vi "Run Test - Pause Condition (SubVI).vi"(8 "error in (no error)":errorcluster, 11 "Cluster in":T1 {"M Event" items=["Stop", "Running", "PID", "Up Limit", "Down Limit", "Load Limit"]; "Test Type" items=["Please Select", "Triaxial Shear", "Triaxial UU", "Shearbox", "Permeability", "Consolidation (Stepped Loading)/Swelling", "Saturation (Incremental)", "User Defined", "UCT", "Isotropic Consolidation", "Swelling Pressure"]; "Data"."Test Type" items=["Please Select", "Triaxial Shear", "Triaxial UU", "Shearbox", "Permeability", "Consolidation (Stepped Loading)/Swelling", "Saturation (Incremental)", "User Defined", "UCT", "Isotropic Consolidation", "Swelling Pressure"]}) -> (0 "error out":errorcluster, 3 "Cluster out":T1 {"M Event" items=["Stop", "Running", "PID", "Up Limit", "Down Limit", "Load Limit"]; "Test Type" items=["Please Select", "Triaxial Shear", "Triaxial UU", "Shearbox", "Permeability", "Consolidation (Stepped Loading)/Swelling", "Saturation (Incremental)", "User Defined", "UCT", "Isotropic Consolidation", "Swelling Pressure"]; "Data"."Test Type" items=["Please Select", "Triaxial Shear", "Triaxial UU", "Shearbox", "Permeability", "Consolidation (Stepped Loading)/Swelling", "Saturation (Incremental)", "User Defined", "UCT", "Isotropic Consolidation", "Swelling Pressure"]})   [LabVIEW 2019]
uses:
  Controls/RunTest - Data Structure.ctl
  Controls/Test Panel - Data Structure.ctl
  Controls/Station - Test Type.ctl
  <vilib>/Utility/miscctls.llb/LVRowAndColumnTypeDef.ctl
  Controls/RunTest - Calculate Data.ctl
  <vilib>/httpClient/ClientHandle.ctl
  Controls/RunTest - Start Condition.ctl
  Controls/RunTest - Stop Condition.ctl
  Controls/UDP - Event.ctl
  Controls/RunTest - State.ctl
  Controls/UDP - Command.ctl
  <vilib>/httpClient/LabVIEWHTTPClient.lvlib
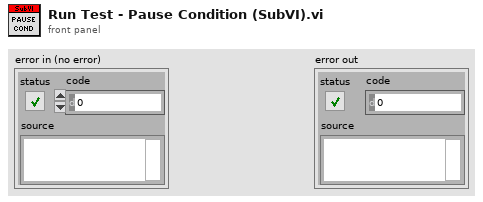
[diagram p1: front panel]
types:
  T1 = typedef "RunTest - Data Structure.ctl" = cluster{"Test Plan":string[], "PlanRow":i32, "Device Name":string[], "Timeout":i32, "Start?":bool, "Pause?":bool, "IP Address":string[], "LogRow":i32, "Logtype":u16, "Log Elapse":sgl, "Data":T2, "Stop log?":bool, "tdms":refnum<k34>, "Sensor Data":sgl[], "Start time":timestamp, "Prev Log Elapse":u32, "Plot":u16, "X-Axis":u16[], "Y-Axis":u16[], "XY":cluster{"X":dbl, "Y":dbl}[][], "End Stage?":bool, "1run":bool, "Condition":u16[], "Start Con":bool, "Log Con":bool, "Stop Con":bool, "Start Elapse":dbl, "Start Load":dbl, "Motor":i32, "StartRow":i32, "number log":i32, "Dir":bool, "Start time test":timestamp, "Auto":bool, "Check return?":bool, "Inv":cluster{"M":i32[], "Bool":bool[]}, "tdms temp":refnum<k34>, "Zero?":bool, "Plot Timer":dbl, "1st Run":bool, "TDMS Path":path, "MaxLoad":dbl, "Log Timer":sgl[], "Test Type":T3, "Log Sensor":string[], "Save?":bool, "1st Log":bool, "Y-Axis 2":u16[], "On Y-Axis 2":bool, "Decimal":u8[], "Init":cluster{"PWP TS":sgl, "Load TS":sgl, "Volume TS":sgl, "Disp TS":sgl, "CP":sgl, "Vol In":sgl, "Vol Out":sgl, "Load UCT":sgl, "Disp UCT":sgl, "PWP Sat":sgl, "CP Sat":sgl, "Volume IsoCons":sgl, "PWP IsoCons":sgl, "PWP TUU":sgl, "Load TUU":sgl, "Volume TUU":sgl, "Disp TUU":sgl, "Load Cons":sgl, "Disp Cons":sgl, "Volume Sat":sgl, "Vertical Load SB":sgl, "Vertical Disp SB":sgl, "H Disp SB":sgl, "H Load SB":sgl}, "Calc":T5, "Device Index":i32[], "Channel Index":i32[], "http ref":T6, "fileid":string, "Step Cons":cluster{"V Stress":sgl, "H Settlement":sgl}, "RunTest":bool, "Graph Last":i32, "Init?":bool, "Datalog":bool[], "Start":T7, "Stop":T8, "Running?":bool, "StartTime":dbl, "Log Prev Time":dbl, "KeyName":string[], "Test RunTime":dbl, "Log Prev Axial":dbl, "M Event":T9[], "Last Log":bool, "popup":bool, "PreStart UU":bool, "PreStart Sat":bool}
  T2 = typedef "Test Panel - Data Structure.ctl" = cluster{"Station":string, "Sample ID":string, "Job No":string, "Job Description":string, "Filename":string, "Test Type":T3, "Speciment No":string, "Depth":string, "Height":string, "Diameter/Length":string, "Weight":string, "Test Parameter":string, "Station[]":string[], "Edit Pos":T4, "Edit Pos Prev":T4, "Area":string, "Path":string}
  T3 = typedef "Station - Test Type.ctl" = u16
  T4 = typedef "LVRowAndColumnTypeDef.ctl" = cluster{"Row":i32, "Column":i32}
  T5 = typedef "RunTest - Calculate Data.ctl" = cluster{"TS":cluster{"Change PWP":sgl, "Change Vol":sgl, "Axial Load":sgl, "CiL":sgl, "Deviator":sgl, "Axial Strain":sgl, "MaxDeviator":sgl}, "TUU":cluster{"Change PWP":sgl, "Axial Load":sgl, "CiL":sgl, "Deviator":sgl, "Axial Strain":sgl, "MaxDeviator":sgl}, "Sat":cluster{"B Value":sgl, "PWP Diss":sgl, "CPP":sgl, "CV":sgl}, "Per":cluster{"Change Vol In":sgl, "Change Vol Out":sgl, "Mean Vol":sgl, "Gradient Pressure":sgl, "Outlet Flow":sgl, "Inlet Flow":sgl, "I X1":sgl, "I X2":sgl, "I Y1":sgl, "I Y2":sgl, "O X1":sgl, "O X2":sgl, "O Y1":sgl, "O Y2":sgl}, "Step Cons":cluster{"V Stress":sgl, "H Settlement":sgl, "Total H Settle":sgl, "Prev Total H":sgl}, "UCT":cluster{"ALC":sgl, "H Change":sgl, "Deviator":sgl, "Axial Strain":sgl, "V Stress":sgl, "MaxDeviator":sgl}, "ISO Cons":cluster{"CPP":sgl, "PWP Diss":sgl, "CV":sgl}, "SB":cluster{"Speci LenC":sgl, "Shear Strain":sgl, "H LC":sgl, "Normal Stress":sgl, "Shear Stress":sgl, "MaxShear":sgl}}
  T6 = typedef "LabVIEWHTTPClient.lvlib/ClientHandle.ctl" = refnum<k1>
  T7 = typedef "RunTest - Start Condition.ctl" = cluster{"Cons":cluster{"VS":dbl, "Delay":bool, "No Delay":dbl}, "Sat":cluster{"CP":dbl, "BP":dbl, "StartBP":bool, "Target CP":bool, "Target BP":bool}, "Iso":cluster{"BP":dbl}, "TS":cluster{"SS":dbl, "Engage":bool, "ES":dbl, "LC":dbl, "PreStart":bool, "Trig SS":bool, "Drain":dbl}, "TUU":cluster{"SS":dbl, "Engage":bool, "ES":dbl, "LC":dbl, "PreStart":bool, "Trig SS":bool, "CP":dbl, "Delay Value":dbl, "Delay":bool, "CP PID":bool}, "UCT":cluster{"SS":dbl, "Engage":bool, "ES":dbl, "LC":dbl, "PreStart":bool, "Trig SS":bool}, "Enable?":bool, "SB":cluster{"SS":dbl, "Engage":bool, "ES":dbl, "LC":dbl, "PreStart":bool, "Trig SS":bool, "VS":dbl, "Delay Value":dbl, "Delay":bool, "VS PID":bool}, "Perm":cluster{"DP":dbl}}
  T8 = typedef "RunTest - Stop Condition.ctl" = cluster{"Cons":cluster{"Select":i32, "Disp":dbl, "Time":dbl, "Time2":dbl, "Disp 2":dbl, "Time Cond":dbl, "Last Disp":dbl, "Swell":bool}, "Sat":cluster{"Select":i32, "PP":dbl, "Time":dbl, "VC":dbl, "Time2":dbl, "Time Cond":dbl, "Last PP":dbl, ".B":bool, "B":dbl, "Last Vc":dbl, "Time Cond 2":dbl, "Time3":dbl, "Time Cond 3":dbl}, "Iso":cluster{"PP":dbl, "Time":dbl, "VC":dbl, "Time2":dbl, "Time Cond":dbl, "Last Vc":dbl, ".PP":bool, "Time Cond 2":dbl, "Select":i32}, "TS":cluster{"Axial":dbl, ".MaxDev":bool, "MaxDev Value":dbl, "Return":bool, "Reset":bool, "Prev Time":dbl, "PostStop Run":bool, "CP Stop":bool, "BP Stop":bool, "PostStop Trig":bool, "Reset Value":dbl, "BPTrig":bool, "CPTrig":bool, "VLCTrig":bool}, "TUU":cluster{"Axial":dbl, ".MaxDev":bool, "MaxDev Value":dbl, "Return":bool, "Reset":bool, "Prev Time":dbl, "PostStop Run":bool, "CP Stop":bool, "BP Stop":bool, "PostStop Trig":bool, "Reset Value":dbl, "BPTrig":bool, "CPTrig":bool, "VLCTrig":bool}, "UCT":cluster{"Axial":dbl, ".MaxDev":bool, "MaxDev Value":dbl, "Return":bool, "Reset":bool, "Prev Time":dbl, "PostStop Run":bool, "CP Stop":bool, "BP Stop":bool, "PostStop Trig":bool}, "Enable?":bool, "SB":cluster{"Shear":dbl, ".MaxShear":bool, "MaxShear Value":dbl, "Return":bool, "Reset":bool, "Prev Time":dbl, "PostStop Run":bool, "CP Stop":bool, "BP Stop":bool, "PostStop Trig":bool, "Reset Value":dbl, "BPTrig":bool, "CPTrig":bool, "VLCTrig":bool}, "Perm":cluster{"Max Time":bool, "Reset":bool, "PostStop Run":bool, "Ratio":bool, "Reset Value":dbl, "Time":dbl, "RatioTime":dbl, "RatioMore":dbl, "RatioLess":dbl, "Time Cond":dbl, "Time Cond 2":dbl, "Prev IF":dbl, "Prev OF":dbl, "PostStop Trig":bool, "BP Trig":bool, "DP Stop":bool, "BP Stop":bool, "CP Stop":bool, "CP Trig":bool}, "SP":cluster{".Max Time":bool, ".Time":bool, "Time":dbl, "MaxTime":dbl, "Time Cond":dbl, "Max Time Cond":dbl, "Stress":dbl}}
  T9 = typedef "UDP - Event.ctl" = u16
  T10 = enum32{"Please Select", "Triaxial Shear", "Triaxial UU", "Shearbox", "Permeability", "Consolidation", "Saturation", "User Defined", "UCT", "Iso Consolidation"}
  T11 = typedef "UDP - Command.ctl" = enum16{"Stop", "Jog Up", "Jog Down", "Ramp Up", "Ramp Down", "PID Target", "PID Ramp", "Disp Run", "Read Ch Data", "Zero Channel", "Zero Disp", "Read Sensor", "Write Sensor", "Read ADC", "Write ADC", "Read PID", "Write PID", "Read Test", "Write Test", "Read System", "Write System", "Read Datalog", "Read Datalog Sensor"}
  T12 = typedef "RunTest - State.ctl" = enum16{"Load Testfile", "Notifier", "Init", "Idle", "Load", "Read DB", "Run", "Pause", "Stop", "Check Start", "Check Stop", "Check Post Stop", "Check Log", "EndStage", "Data View", "Display", "Graph", "Graph Old", "Close", "Stop PID", "Check Limit", "Auto", "Up", "Log", "Zero", "Machine Control", "Save Report"}
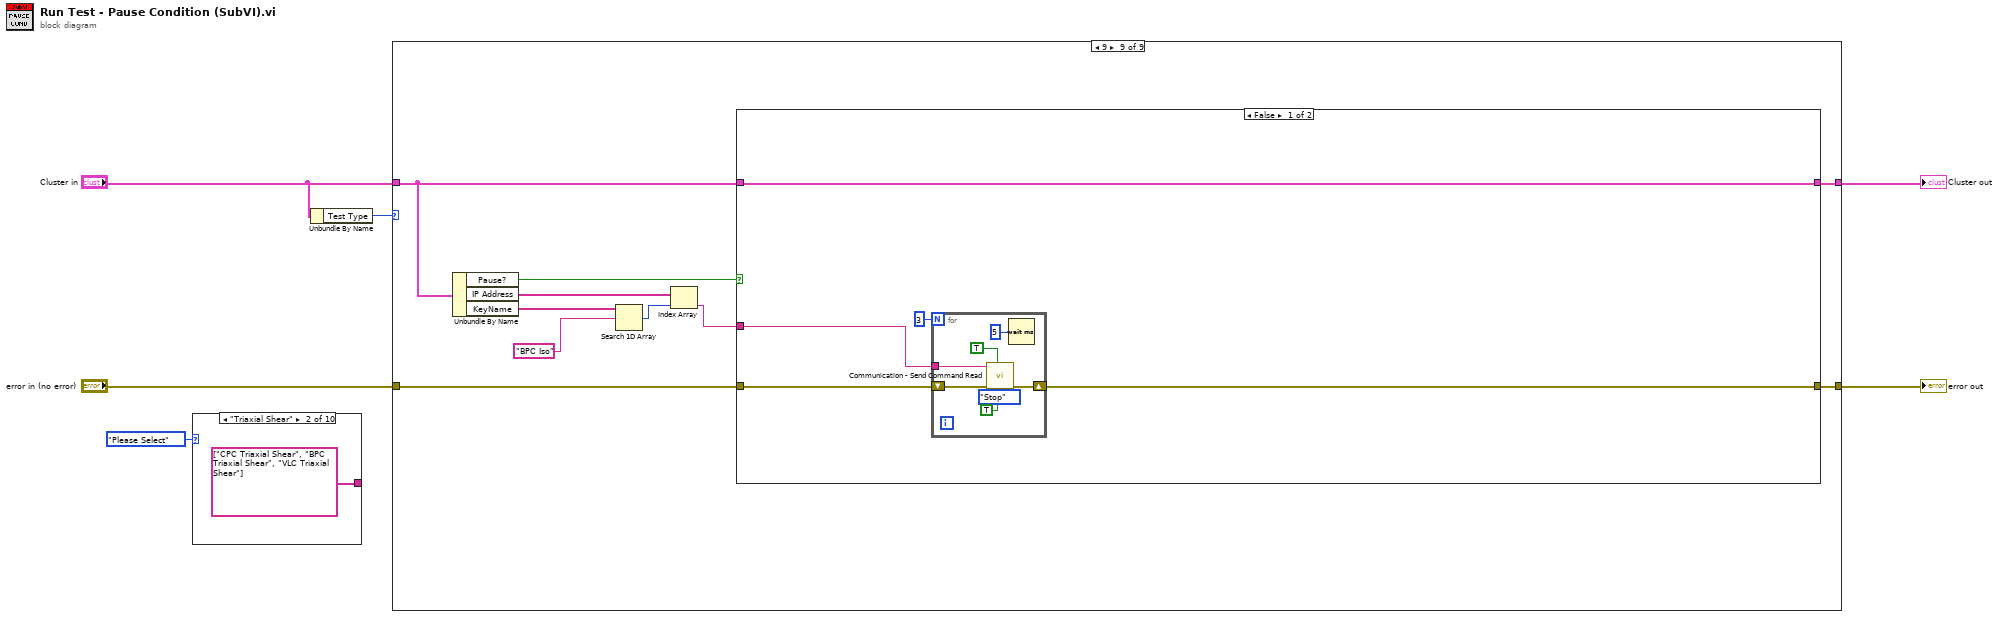
[diagram p0: block diagram]
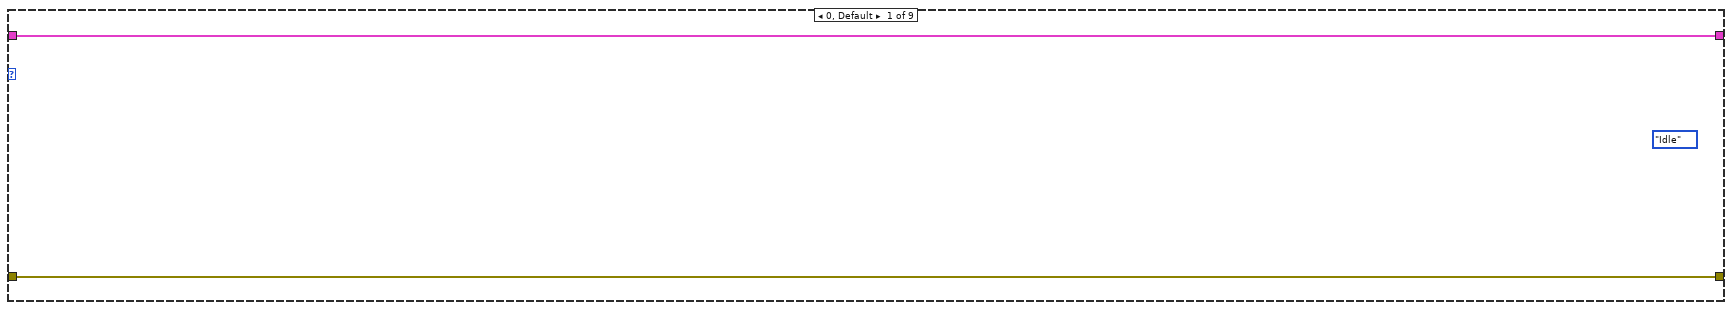
[diagram p2: hidden frame]
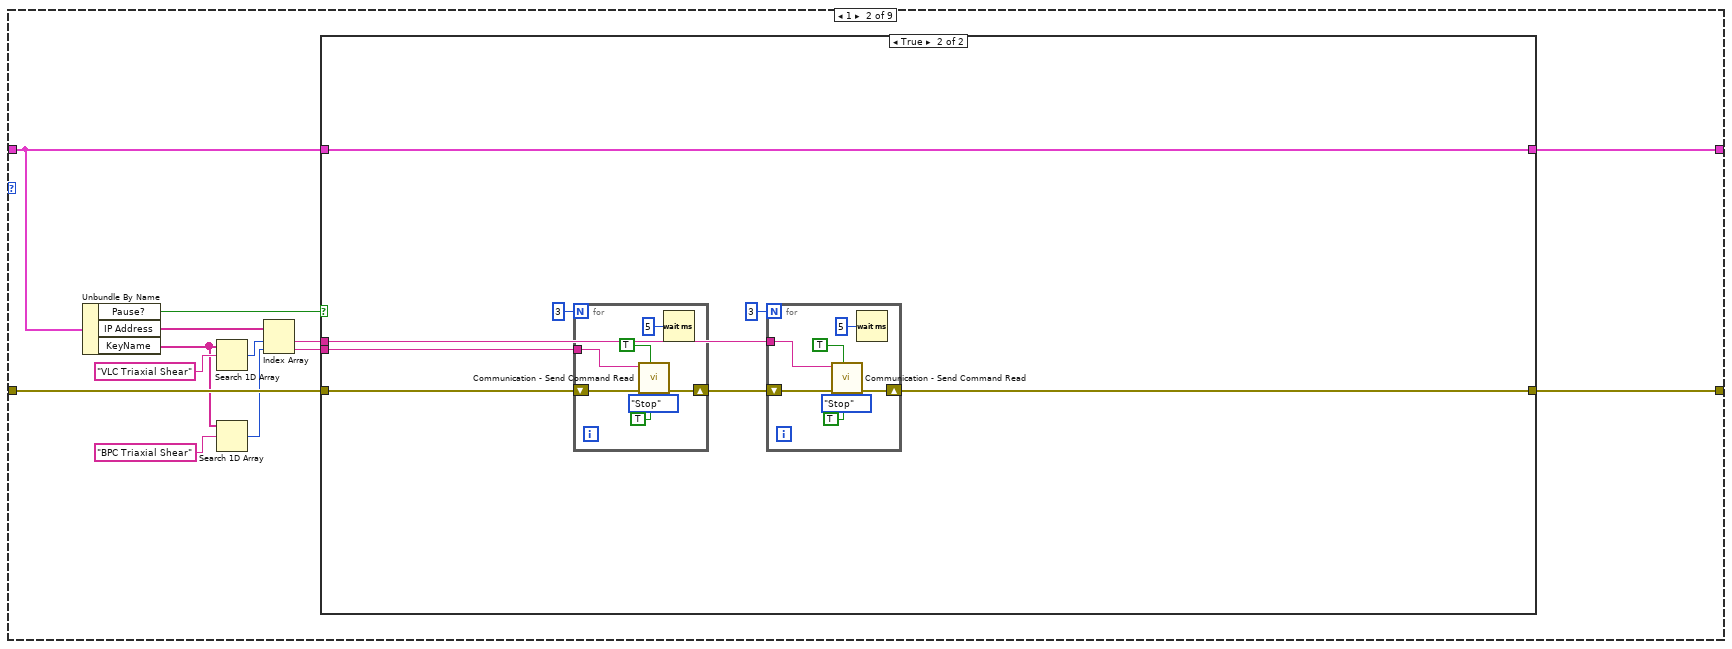
[diagram p3: hidden frame]
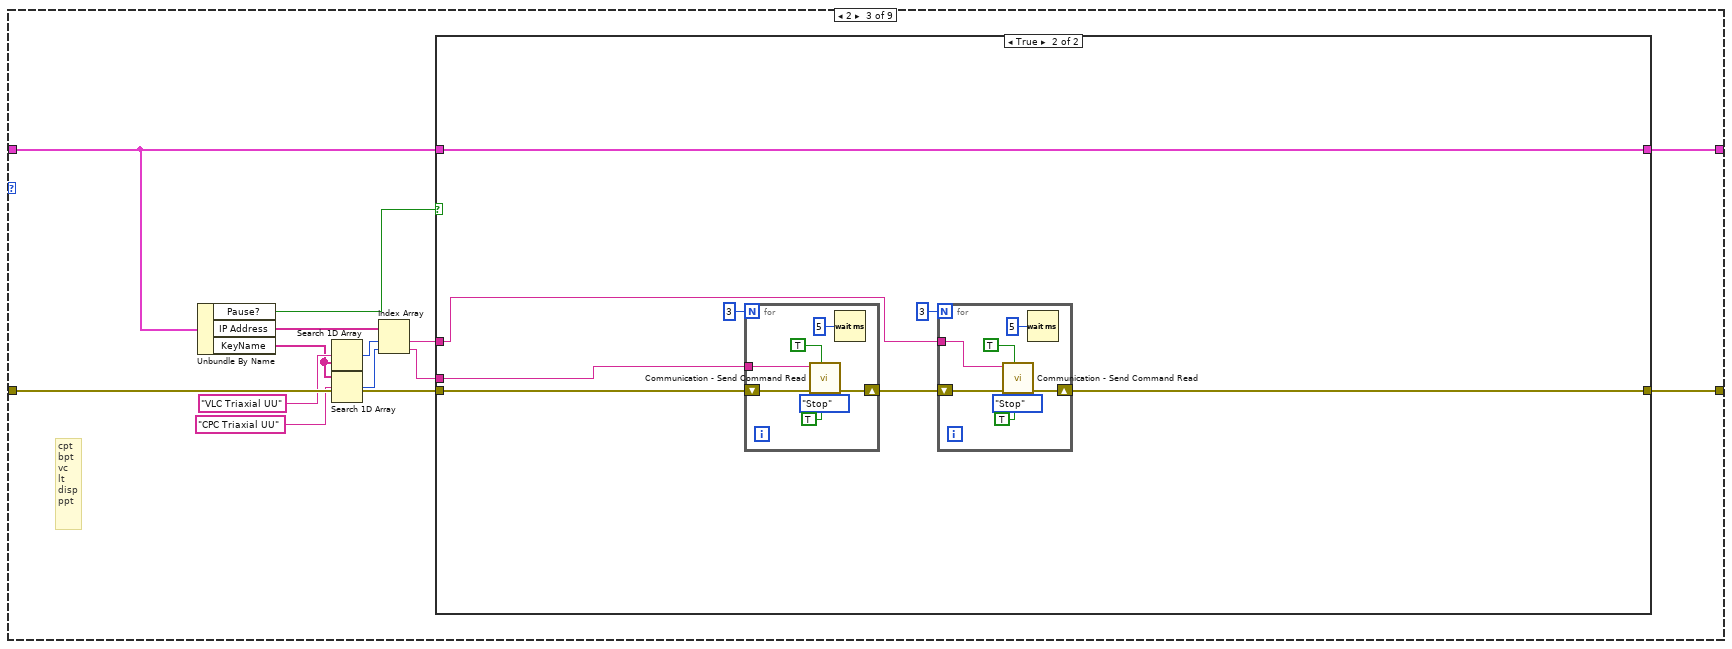
[diagram p5: hidden frame]
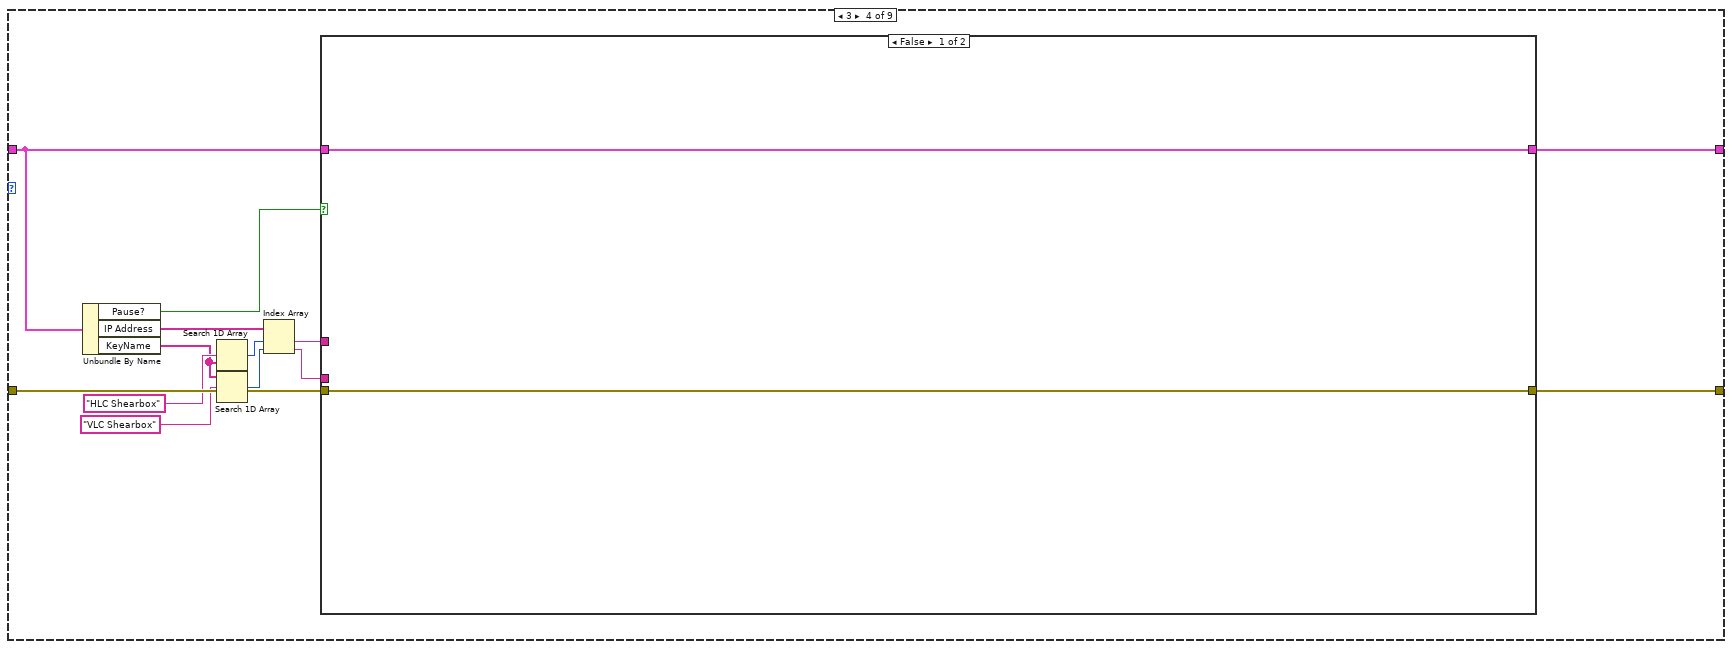
[diagram p7: hidden frame]
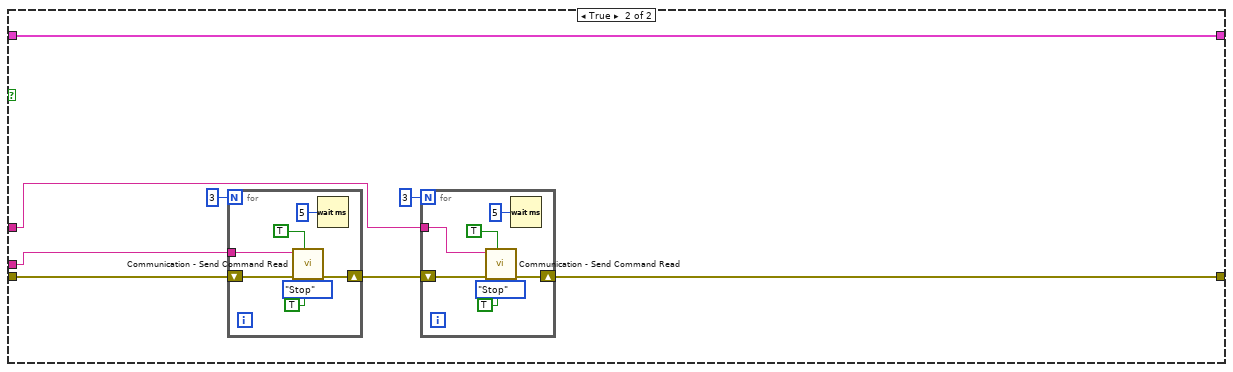
[diagram p8: hidden frame]
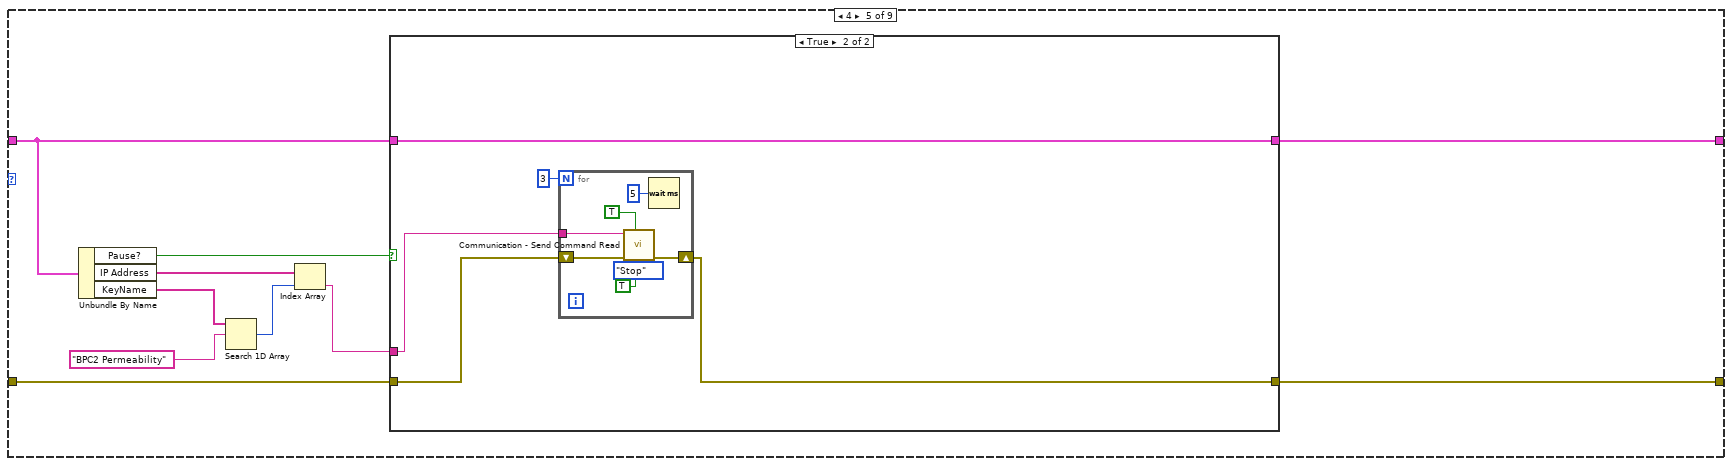
[diagram p9: hidden frame]
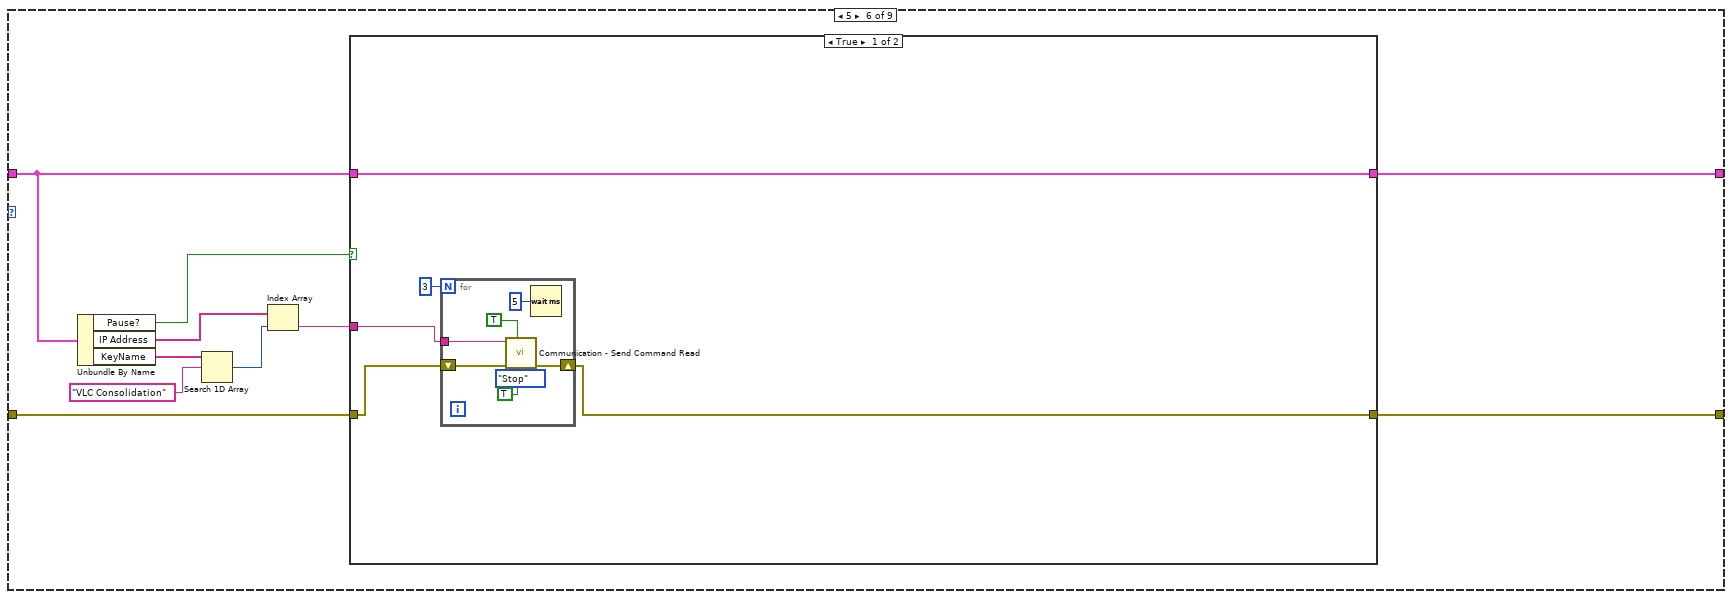
[diagram p11: hidden frame]
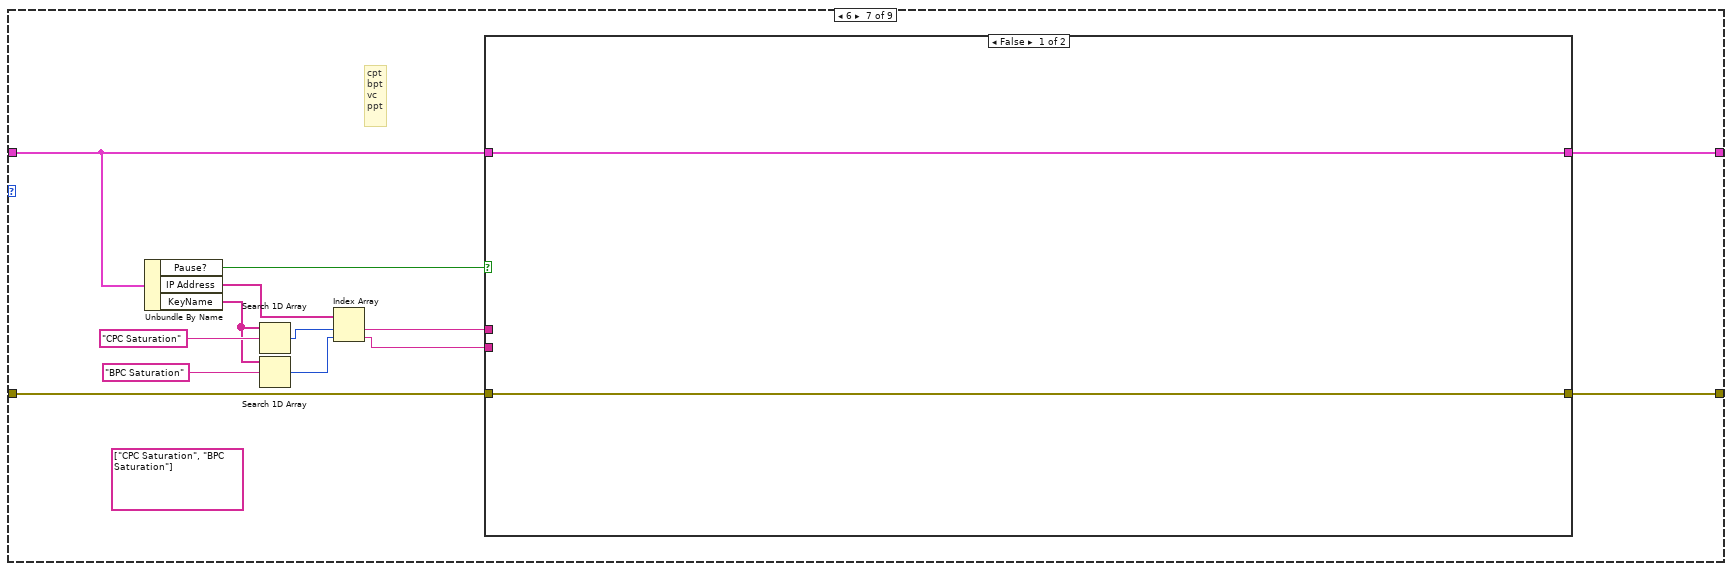
[diagram p13: hidden frame]
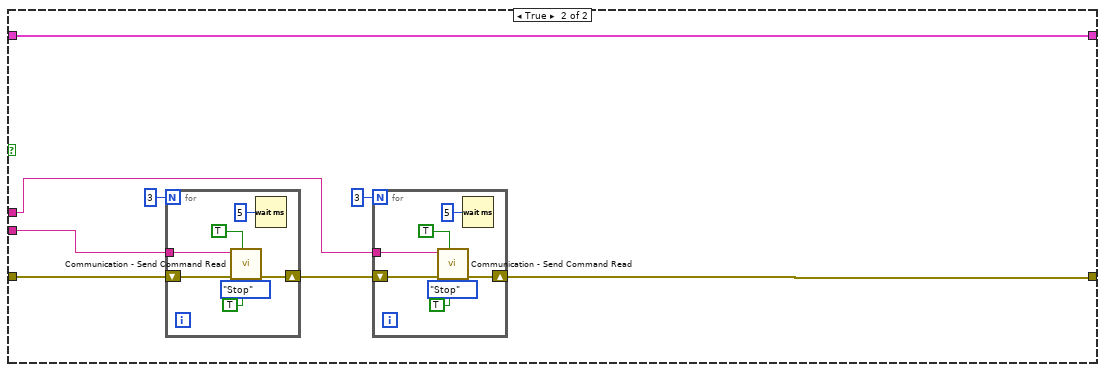
[diagram p14: hidden frame]
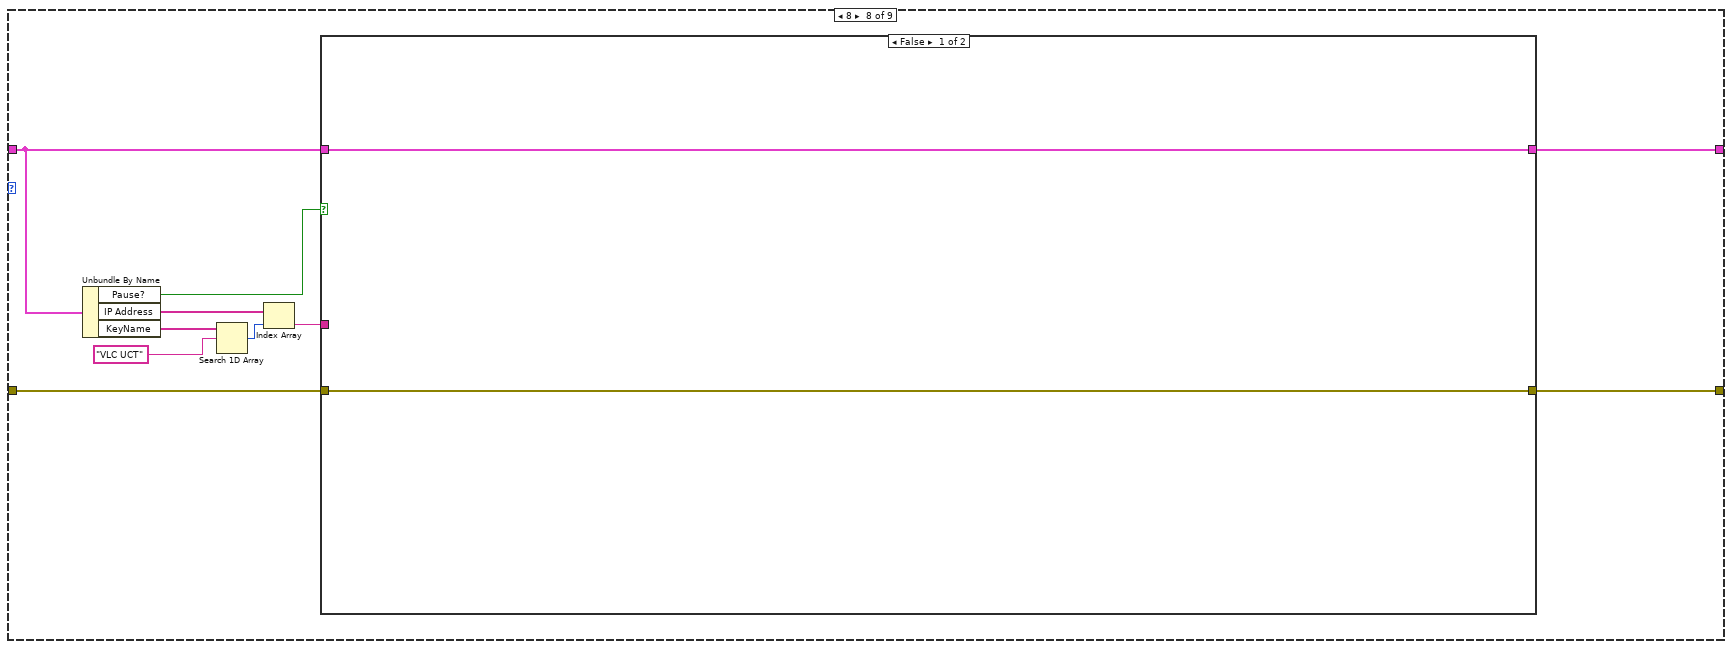
[diagram p15: hidden frame]
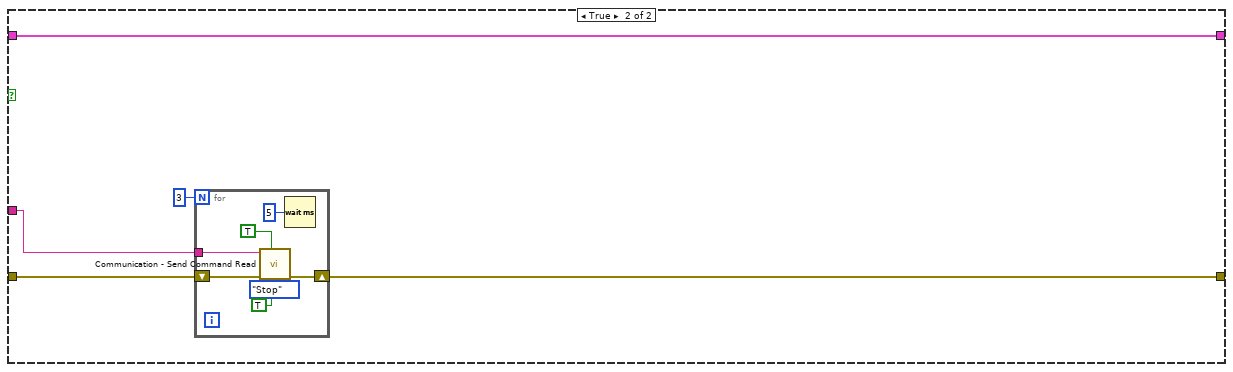
[diagram p16: hidden frame]
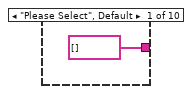
[diagram p18: hidden frame]
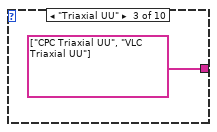
[diagram p19: hidden frame]
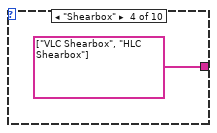
[diagram p20: hidden frame]
diagram:
  n1 = case shown="\"Triaxial Shear\"" T10."Please Select" ("Sub Tab") {
    tunnel: [string[] [] string[] ["CPC Triaxial Shear", "BPC Triaxial Shear", "VLC Triaxial Shear"] string[] ["CPC Triaxial UU", "VLC Triaxial UU"] string[] ["VLC Shearbox", "HLC Shearbox"] string[] ["CPC Permeability", "BPC Permeability", "BPC2 Permeability"] string[] ["VLC Consolidation"] string[] ["CPC Saturation", "BPC Saturation"] string[] ["CPC User Defined", "BPC User Defined", "BPC2 User Defined", "VLC User Defined", "HLC User Defined"] string[] ["VLC UCT"] string[] ["CPC Iso", "BPC Iso"]] -> _
    frame "Please Select", Default {
    }
    frame "Triaxial Shear" {
    }
    frame "Triaxial UU" {
    }
    frame "Shearbox" {
    }
    frame "Permeability" {
    }
    frame "Consolidation" {
    }
    frame "Saturation" {
    }
    frame "User Defined" {
    }
    frame "UCT" {
    }
    frame "Iso Consolidation" {
    }
  }
  n2 = Unbundle By Name("Cluster in") -> ("Test Type"=w1:T3)
  n3 = case shown="9" w1 {
    tunnel: [w18 w29 w67 w94 w136 w161 w188 w222 w245] -> w3
    tunnel: "Cluster in" -> [w18 w30 w65 w104 w135 w160 w187 w223 w244]
    tunnel: [w17 w28 w66 w95 w139 w163 w190 w221 w248] -> w5
    tunnel: "error in (no error)" -> [w17 w31 w68 w105 w138 w162 w189 w224 w247]
    frame 0, Default {
      (unwired) RunTest_-_State."Idle"
    }
    frame 1 {
      n4 = Unbundle By Name(w30) -> ("Pause?"=w19:bool, "IP Address"=w26:string[], "KeyName"=w22:string[])
      n5 = Search 1D Array(1D array=w22, element="VLC Triaxial Shear" ("String")) -> (index of element=w27:i32)  [unwired: 1 in]
      n6 = Search 1D Array(1D array=w22, element="BPC Triaxial Shear" ("String")) -> (index of element=w21:i32)  [unwired: 1 in]
      n7 = Index Array(array=w26, index #1=w27, index #2=w21) -> (element #1=w24:string, element #2=w20:string)
      n8 = case shown="True" w19 {
        tunnel: w31 -> [w33 w41]
        tunnel: w30 -> [w32 w40]
        tunnel: [w32 w40] -> w29
        tunnel: [w33 w35] -> w28
        tunnel: w24 -> [_ w34]
        tunnel: w20 -> [_ w39]
        frame False {
        }
        frame True {
          n9 = for {
            N: 3 -> [_]
            tunnel: w39 -> [w50]
            shift-right: [w51] -> w36
            shift-left: w41 -> [w52]
            n10 = call "Communication - Send Command Read.vi"("Fron?"=TRUE, "Bypass?"=TRUE, "error in (no error)"=w52, "Action"=UDP_-_Command."Stop", "Device IP Address"=w50) -> ("error out"=w51:errorcluster)  [unwired: 6 in]
            n11 = Wait (ms)(milliseconds to wait=u32 5) -> ()  [unwired: 1 out]
          }
          n12 = for {
            N: 3 -> [_]
            tunnel: w34 -> [w43]
            shift-right: [w44] -> w35
            shift-left: w36 -> [w45]
            n13 = call "Communication - Send Command Read.vi"("Fron?"=TRUE, "Bypass?"=TRUE, "error in (no error)"=w45, "Action"=UDP_-_Command."Stop", "Device IP Address"=w43) -> ("error out"=w44:errorcluster)  [unwired: 6 in]
            n14 = Wait (ms)(milliseconds to wait=u32 5) -> ()  [unwired: 1 out]
          }
        }
      }
    }
    frame 2 {
      # "cpt\nbpt\nvc\nlt\ndisp\nppt"
      n15 = Unbundle By Name(w65) -> ("Pause?"=w56:bool, "IP Address"=w63:string[], "KeyName"=w60:string[])
      n16 = Search 1D Array(1D array=w60, element="VLC Triaxial UU" ("String")) -> (index of element=w64:i32)  [unwired: 1 in]
      n17 = Search 1D Array(1D array=w60, element="CPC Triaxial UU" ("String")) -> (index of element=w58:i32)  [unwired: 1 in]
      n18 = Index Array(array=w63, index #1=w64, index #2=w58) -> (element #1=w61:string, element #2=w57:string)
      n19 = case shown="True" w56 {
        tunnel: w68 -> [w69 w74]
        tunnel: w65 -> [w70 w78]
        tunnel: [w70 w78] -> w67
        tunnel: [w69 w73] -> w66
        tunnel: w61 -> [_ w71]
        tunnel: w57 -> [_ w72]
        frame False {
        }
        frame True {
          n20 = for {
            N: 3 -> [_]
            shift-right: [w88] -> w75
            shift-left: w74 -> [w89]
            tunnel: w72 -> [w86]
            n21 = call "Communication - Send Command Read.vi"("Fron?"=TRUE, "Bypass?"=TRUE, "error in (no error)"=w89, "Action"=UDP_-_Command."Stop", "Device IP Address"=w86) -> ("error out"=w88:errorcluster)  [unwired: 6 in]
            n22 = Wait (ms)(milliseconds to wait=u32 5) -> ()  [unwired: 1 out]
          }
          n23 = for {
            N: 3 -> [_]
            tunnel: w71 -> [w80]
            shift-right: [w81] -> w73
            shift-left: w75 -> [w82]
            n24 = call "Communication - Send Command Read.vi"("Fron?"=TRUE, "Bypass?"=TRUE, "error in (no error)"=w82, "Action"=UDP_-_Command."Stop", "Device IP Address"=w80) -> ("error out"=w81:errorcluster)  [unwired: 6 in]
            n25 = Wait (ms)(milliseconds to wait=u32 5) -> ()  [unwired: 1 out]
          }
        }
      }
    }
    frame 3 {
      n26 = Unbundle By Name(w104) -> ("Pause?"=w93:bool, "IP Address"=w102:string[], "KeyName"=w99:string[])
      n27 = Search 1D Array(1D array=w99, element="HLC Shearbox" ("String")) -> (index of element=w103:i32)  [unwired: 1 in]
      n28 = Search 1D Array(1D array=w99, element="VLC Shearbox" ("String")) -> (index of element=w97:i32)  [unwired: 1 in]
      n29 = Index Array(array=w102, index #1=w103, index #2=w97) -> (element #1=w100:string, element #2=w96:string)
      n30 = case shown="False" w93 {
        tunnel: w105 -> [w106 w112]
        tunnel: w104 -> [w107 w110]
        tunnel: w100 -> [_ w108]
        tunnel: w96 -> [_ w109]
        tunnel: [w106 w111] -> w95
        tunnel: [w107 w110] -> w94
        frame False {
        }
        frame True {
          n31 = for {
            N: 3 -> [_]
            shift-right: [w125] -> w113
            shift-left: w112 -> [w126]
            tunnel: w109 -> [w123]
            n32 = call "Communication - Send Command Read.vi"("Fron?"=TRUE, "Bypass?"=TRUE, "error in (no error)"=w126, "Action"=UDP_-_Command."Stop", "Device IP Address"=w123) -> ("error out"=w125:errorcluster)  [unwired: 6 in]
            n33 = Wait (ms)(milliseconds to wait=u32 5) -> ()  [unwired: 1 out]
          }
          n34 = for {
            N: 3 -> [_]
            tunnel: w108 -> [w117]
            shift-right: [w118] -> w111
            shift-left: w113 -> [w119]
            n35 = call "Communication - Send Command Read.vi"("Fron?"=TRUE, "Bypass?"=TRUE, "error in (no error)"=w119, "Action"=UDP_-_Command."Stop", "Device IP Address"=w117) -> ("error out"=w118:errorcluster)  [unwired: 6 in]
            n36 = Wait (ms)(milliseconds to wait=u32 5) -> ()  [unwired: 1 out]
          }
        }
      }
    }
    frame 4 {
      n37 = Unbundle By Name(w135) -> ("Pause?"=w137:bool, "IP Address"=w132:string[], "KeyName"=w134:string[])
      n38 = Search 1D Array(1D array=w134, element="BPC2 Permeability" ("String")) -> (index of element=w131:i32)  [unwired: 1 in]
      n39 = Index Array(array=w132, index=w131) -> (element=w130:string)
      n40 = case shown="True" w137 {
        tunnel: [w141 w143] -> w139
        tunnel: w138 -> [w141 w144]
        tunnel: [w140 w146] -> w136
        tunnel: w135 -> [w140 w146]
        tunnel: w130 -> [_ w142]
        frame False {
        }
        frame True {
          n41 = for {
            N: 3 -> [_]
            shift-right: [w149] -> w143
            shift-left: w144 -> [w150]
            tunnel: w142 -> [w147]
            n42 = call "Communication - Send Command Read.vi"("Fron?"=TRUE, "Bypass?"=TRUE, "error in (no error)"=w150, "Action"=UDP_-_Command."Stop", "Device IP Address"=w147) -> ("error out"=w149:errorcluster)  [unwired: 6 in]
            n43 = Wait (ms)(milliseconds to wait=u32 5) -> ()  [unwired: 1 out]
          }
        }
      }
    }
    frame 5 {
      n44 = Unbundle By Name(w160) -> ("Pause?"=w154:bool, "IP Address"=w157:string[], "KeyName"=w159:string[])
      n45 = Search 1D Array(1D array=w159, element="VLC Consolidation" ("String")) -> (index of element=w156:i32)  [unwired: 1 in]
      n46 = Index Array(array=w157, index=w156) -> (element=w155:string)
      n47 = case shown="True" w154 {
        tunnel: [w164 w176] -> w163
        tunnel: w162 -> [w166 w176]
        tunnel: [w168 w177] -> w161
        tunnel: w160 -> [w168 w177]
        tunnel: w155 -> [w165 _]
        frame True {
          n48 = for {
            N: 3 -> [_]
            shift-right: [w171] -> w164
            shift-left: w166 -> [w172]
            tunnel: w165 -> [w169]
            n49 = call "Communication - Send Command Read.vi"("Fron?"=TRUE, "Bypass?"=TRUE, "error in (no error)"=w172, "Action"=UDP_-_Command."Stop", "Device IP Address"=w169) -> ("error out"=w171:errorcluster)  [unwired: 6 in]
            n50 = Wait (ms)(milliseconds to wait=u32 5) -> ()  [unwired: 1 out]
          }
        }
        frame False {
        }
      }
    }
    frame 6 {
      (unwired) string[] ["CPC Saturation", "BPC Saturation"]
      # "cpt\nbpt\nvc\nppt"
      n51 = Unbundle By Name(w187) -> ("Pause?"=w186:bool, "IP Address"=w183:string[], "KeyName"=w182:string[])
      n52 = Search 1D Array(1D array=w182, element="CPC Saturation" ("String")) -> (index of element=w185:i32)  [unwired: 1 in]
      n53 = Search 1D Array(1D array=w182, element="BPC Saturation" ("String")) -> (index of element=w180:i32)  [unwired: 1 in]
      n54 = Index Array(array=w183, index #1=w185, index #2=w180) -> (element #1=w179:string, element #2=w178:string)
      n55 = case shown="False" w186 {
        tunnel: [w191 w196] -> w190
        tunnel: w189 -> [w191 w195]
        tunnel: [w192 w200] -> w188
        tunnel: w187 -> [w192 w200]
        tunnel: w179 -> [_ w194]
        tunnel: w178 -> [_ w193]
        frame False {
        }
        frame True {
          n56 = for {
            N: 3 -> [_]
            shift-right: [w210] -> w197
            shift-left: w195 -> [w211]
            tunnel: w193 -> [w208]
            n57 = call "Communication - Send Command Read.vi"("Fron?"=TRUE, "Bypass?"=TRUE, "error in (no error)"=w211, "Action"=UDP_-_Command."Stop", "Device IP Address"=w208) -> ("error out"=w210:errorcluster)  [unwired: 6 in]
            n58 = Wait (ms)(milliseconds to wait=u32 5) -> ()  [unwired: 1 out]
          }
          n59 = for {
            N: 3 -> [_]
            shift-right: [w203] -> w196
            shift-left: w197 -> [w204]
            tunnel: w194 -> [w201]
            n60 = call "Communication - Send Command Read.vi"("Fron?"=TRUE, "Bypass?"=TRUE, "error in (no error)"=w204, "Action"=UDP_-_Command."Stop", "Device IP Address"=w201) -> ("error out"=w203:errorcluster)  [unwired: 6 in]
            n61 = Wait (ms)(milliseconds to wait=u32 5) -> ()  [unwired: 1 out]
          }
        }
      }
    }
    frame 8 {
      n62 = Unbundle By Name(w223) -> ("Pause?"=w215:bool, "IP Address"=w219:string[], "KeyName"=w218:string[])
      n63 = Search 1D Array(1D array=w218, element="VLC UCT" ("String")) -> (index of element=w220:i32)  [unwired: 1 in]
      n64 = Index Array(array=w219, index=w220) -> (element=w216:string)
      n65 = case shown="False" w215 {
        tunnel: w224 -> [w225 w230]
        tunnel: w223 -> [w226 w227]
        tunnel: [w226 w227] -> w222
        tunnel: [w225 w229] -> w221
        tunnel: w216 -> [_ w228]
        frame False {
        }
        frame True {
          n66 = for {
            N: 3 -> [_]
            shift-right: [w234] -> w229
            shift-left: w230 -> [w235]
            tunnel: w228 -> [w232]
            n67 = call "Communication - Send Command Read.vi"("Fron?"=TRUE, "Bypass?"=TRUE, "error in (no error)"=w235, "Action"=UDP_-_Command."Stop", "Device IP Address"=w232) -> ("error out"=w234:errorcluster)  [unwired: 6 in]
            n68 = Wait (ms)(milliseconds to wait=u32 5) -> ()  [unwired: 1 out]
          }
        }
      }
    }
    frame 9 {
      n69 = Unbundle By Name(w244) -> ("Pause?"=w246:bool, "IP Address"=w240:string[], "KeyName"=w241:string[])
      n70 = Search 1D Array(1D array=w241, element="BPC Iso" ("String")) -> (index of element=w243:i32)  [unwired: 1 in]
      n71 = Index Array(array=w240, index=w243) -> (element=w239:string)
      n72 = case shown="False" w246 {
        tunnel: [w250 w261] -> w248
        tunnel: w247 -> [w251 w261]
        tunnel: [w253 w262] -> w245
        tunnel: w244 -> [w253 w262]
        tunnel: w239 -> [w249 _]
        frame False {
          n73 = for {
            N: 3 -> [_]
            shift-right: [w256] -> w250
            shift-left: w251 -> [w257]
            tunnel: w249 -> [w254]
            n74 = call "Communication - Send Command Read.vi"("Fron?"=TRUE, "Bypass?"=TRUE, "error in (no error)"=w257, "Action"=UDP_-_Command."Stop", "Device IP Address"=w254) -> ("error out"=w256:errorcluster)  [unwired: 6 in]
            n75 = Wait (ms)(milliseconds to wait=u32 5) -> ()  [unwired: 1 out]
          }
        }
        frame True {
        }
      }
    }
  }
  "error out" <- w5
  "Cluster out" <- w3
